vi "LogStatus.vi"(9 "text":string, 11 "file path":path) -> ()   [LabVIEW 2024, in "LVarex.lvlib"]
uses:
  LVarex.lvlib
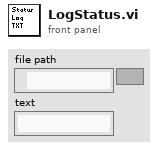
[diagram p1: front panel]
types:
  T1 = enum16{"open", "replace", "create", "open or create", "replace or create", "replace or create with confirmation"}
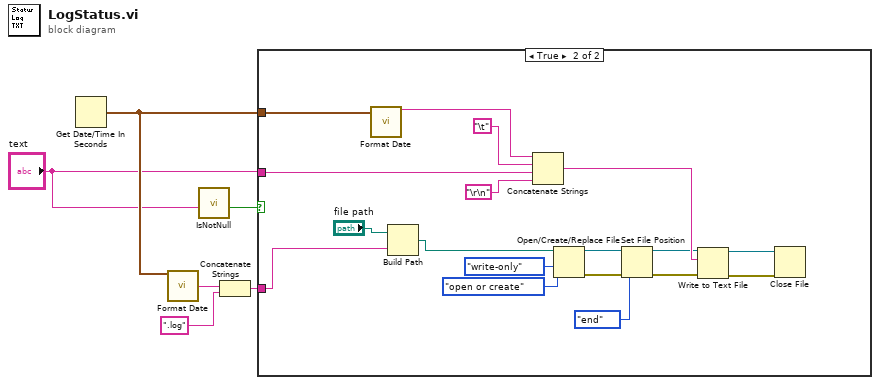
[diagram p0: block diagram]
diagram:
  n1 = Get Date/Time In Seconds() -> (seconds since 1Jan1904=w6:timestamp)
  n2 = call "Format Date.vi"("Time Stamp In"=w6) -> ("Filename Date Out"=w5:string)  [unwired: 10 in, 4 out]
  n3 = call "IsNotNull.vi"("String In"="text") -> ("Boolean Out"=w2:bool)  [unwired: 10 in]
  n4 = Concatenate Strings(w5, ".log") -> (w3:string)
  n5 = case shown="True" w2 {
    tunnel: "text" -> [_ w18]
    tunnel: w6 -> [_ w8]
    tunnel: w3 -> [_ w7]
    frame False {
    }
    frame True {
      n6 = call "Format Date.vi"("Time Stamp In"=w8) -> ("Formatted DateTime Out"=w9:string)  [unwired: 10 in, 4 out]
      n7 = Build Path(base path="file path", name or relative path=w7) -> (appended path=w19:path)
      n8 = Concatenate Strings(w9, "\t", w18, "\r\n") -> (w17:string)
      n9 = Open/Create/Replace File(file path (use dialog)=w19, operation (0:open)=T1."open or create", access (0:read/write)=enum16{"read/write", "read-only", "write-only"}."write-only") -> (refnum out=w14:refnum<file>, error out=w13:errorcluster)  [unwired: 3 in, 1 out]
      n10 = Set File Position(refnum=w14, from (0:start)=enum16{"start", "end", "current"}."end", error in=w13) -> (refnum out=w11:refnum<file>, error out=w10:errorcluster)  [unwired: 1 in]
      n11 = Write to Text File(file (use dialog)=w11, text=w17, error in=w10) -> (refnum out=w22:refnum<file>, error out=w21:errorcluster)  [unwired: 1 in, 1 out]
      n12 = Close File(refnum=w22, error in=w21) -> ()  [unwired: 2 out]
    }
  }
